vi "orderDefPos.vi"(8 "error in (no error)":errorcluster, 9 "Def Positions":dbl[][](array[numeric]) format="%#_13g", 10 "Game":refnum<class "Game.lvclass">, 11 "Utilities in":refnum<class "Utilities.lvclass">) -> (0 "error out":errorcluster, 2 "Ordered Positions":dbl[][](array[numeric]), 3 "Utilities out":refnum<class "Utilities.lvclass">)   [LabVIEW 2023, in "Utilities.lvclass"]
uses:
  Utilities.lvclass
  Game_class/Game.lvclass
  Game_class/Game.lvclass/Game.ctl
  127db9f2-95dc-497e-9bb6-d2ce9a48d1cd.vi
  Game_class/Read FieldRef.vi
  <vilib>/Array/Sort 2D Array - Pop Stack.vi
  <vilib>/Array/Sort 2D Array - Push Stack.vi
  127db9f2-95dc-497e-9bb6-d2ce9a48d1cd.vi/269d4b3b-47f5-49e3-8884-44851e4dd9d5.vi
  127db9f2-95dc-497e-9bb6-d2ce9a48d1cd.vi/6d99389c-673d-4efb-bf33-19b32bcf4cf8.vi
  Field_class/Field.lvclass
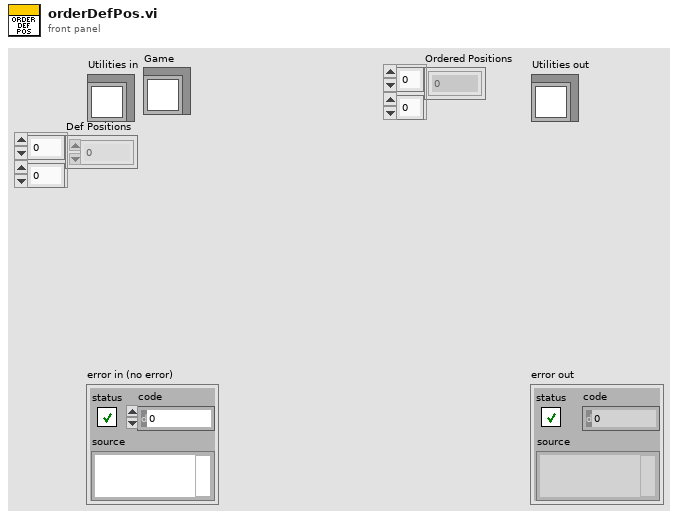
[diagram p1: front panel]
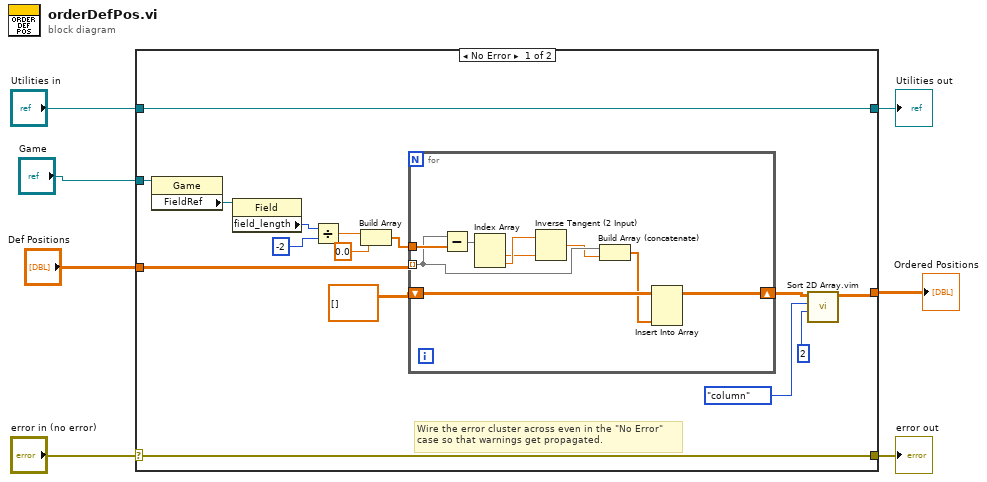
[diagram p0: block diagram]
diagram:
  n1 = case shown="No Error" "error in (no error)" {
    selector: "error in (no error)" -> [w21 w34]
    tunnel: [w21 w34] -> w6
    tunnel: [w22 w33] -> w4
    tunnel: "Utilities in" -> [w22 w33]
    tunnel: "Def Positions" -> [w11 w32]
    tunnel: "Game" -> [w20 _]
    tunnel: [w14 w32] -> w1
    frame No Error {
      # "Wire the error cluster across even in the \"No Error\"\ncase so that warnings get propagated."
      n2 = property class="Game"(reference=w20) -> ("FieldRef"=w19:refnum<class "Field.lvclass">)  [unwired: 1 in, 2 out]
      n3 = property class="Field"(reference=w19) -> ("field_length"=w8:i32)  [unwired: 1 in, 2 out]
      n4 = Divide(x=w8, y=-2) -> (x/y=w17:dbl)
      n5 = Build Array(w17, 0.0 ("element")) -> (w15:dbl[])
      n6 = for {
        tunnel: w11 -> [w27] mode=indexing
        tunnel: w15 -> [w31]
        shift-right: [w25] -> w9
        shift-left: dbl[][] [] -> [w24]
        n7 = Subtract(x=w27, y=w31) -> (x-y=w30:dbl[])
        n8 = Index Array(array=w30) -> (element #1=w28:dbl, element #2=w29:dbl)  [unwired: 2 in]
        n9 = Inverse Tangent (2 Input)(1:w28, 2:w29) -> (0:w26:dbl)
        n10 = Build Array (concatenate)(w27, w26) -> (w23:dbl[])
        n11 = Insert Into Array(array=w24, new element=w23) -> (w25:dbl[][])  [unwired: 2 in]
      }
      n12 = call "Sort 2D Array.vim"("index"=2, "dimension to index (column)"=enum16{"column", "row"}."column", "2D array"=w9) -> ("sorted 2D array"=w14:dbl[][])  [unwired: 7 in, 1 out]
    }
    frame Error {
    }
  }
  "error out" <- w6
  "Utilities out" <- w4
  "Ordered Positions" <- w1
